vi "Create Groups.vi"(8 "error in (no error)":errorcluster, 10 "Framework Configuration":refnum<class "Framework Configuration.lvclass">, 11 "Framework in":refnum<class "Framework.lvclass">) -> (0 "error out":errorcluster, 2 "Transfer Groups":refnum<class "Transfer Group.lvclass">[](array[class]), 3 "Framework out":refnum<class "Framework.lvclass">)   [LabVIEW 2017, in "DSF Core.lvlib" / "Framework.lvclass"]
uses:
  Framework.lvclass
  Configuration/Core/Framework/Framework Configuration.lvclass
  Transfer Group/Transfer Group.lvclass
  Configuration/Core/Framework/Framework Configuration.lvclass/Framework Configuration.ctl
  Configuration/Core/Plugin/Plugin Configuration.lvclass/Plugin Configuration.ctl
  Configuration/Core/Thread/Thread Configuration.lvclass/Thread Configuration.ctl
  Buffer/Buffer.lvclass
  C:/Program Files (x86)/National Instruments/LabVIEW 2017/vi.lib/NI/Memory Manager/Classes/Pointer/Pointer.lvclass
  Configuration/Core/Group/Group Configuration.lvclass/Group Configuration.ctl
  <vilib>/NI/Memory Manager/Classes/Pointer/Pointer.lvclass/Pointer.ctl
  Transfer Group/Transfer Offsets.ctl
  <vilib>/NI/Memory Manager/Classes/Pointer/Set Size.vi
  <vilib>/NI/Memory Manager/Classes/Pointer/Set Address.vi
  <vilib>/NI/Memory Manager/Classes/Pointer/Check Null Pointer.vi
  <vilib>/NI/Memory Manager/Classes/Pointer/Set Internal.vi
  <vilib>/NI/Memory Manager/Classes/Pointer/Errors.vi
  <vilib>/NI/Memory Manager/Classes/Pointer/Null Pointer.vi
  <vilib>/NI/Memory Manager/Classes/Pointer/Is Null.vi
  <vilib>/NI/Memory Manager/Classes/Pointer/Create Error.vi
  <vilib>/NI/Memory Manager/Classes/Pointer/Get Address.vi
  <vilib>/NI/Memory Manager/Constants/Constants.vi
  <vilib>/NI/Memory Manager/Constants/Library Name.vi
  <vilib>/NI/Memory Manager/Classes/Pointer/Pointer Error Info.vi
  <vilib>/NI/Memory Manager/Constants/Pointer Class Name.vi
  <vilib>/NI/Memory Manager/VIs/New Error Cluster.vi
  <vilib>/NI/Memory Manager/VIs/New Error Cluster (512B).vi
  <vilib>/NI/Memory Manager/VIs/Set Error Status.vi
  <vilib>/NI/Memory Manager/VIs/Set Error Code.vi
  <vilib>/NI/Memory Manager/VIs/Set Error Source.vi
  <vilib>/NI/Memory Manager/VIs/Write String to Source.vi
  Configuration/Core/Group/Group Configuration.lvclass
  Configuration/Core/Transfer/Transfer Configuration.lvclass
  Configuration/Core/Plugin/Plugin Configuration.lvclass
  Configuration/Core/Thread/Thread Configuration.lvclass
  <vilib>/NI/Memory Manager/Classes/Pointer/Pointer.lvclass
  Buffers/Buffers.lvclass
  Transfer/Transfer.lvclass
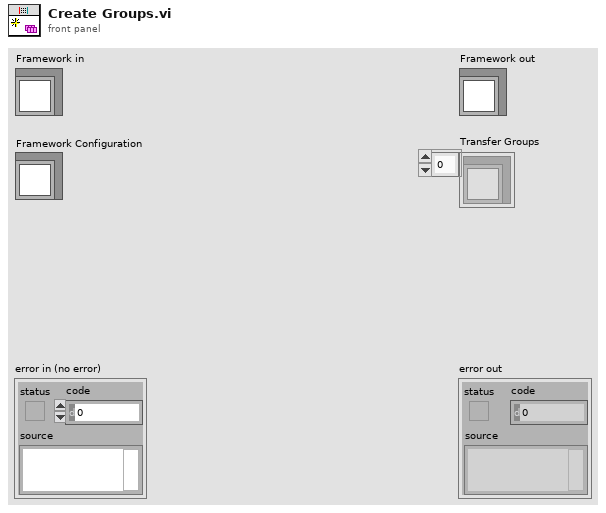
[diagram p1: front panel]
types:
  T1 = typedef "DSF Core.lvlib/Transfer Group.lvclass/Transfer Offsets.ctl" = cluster{"string offset":u64, "engine offset":u64}
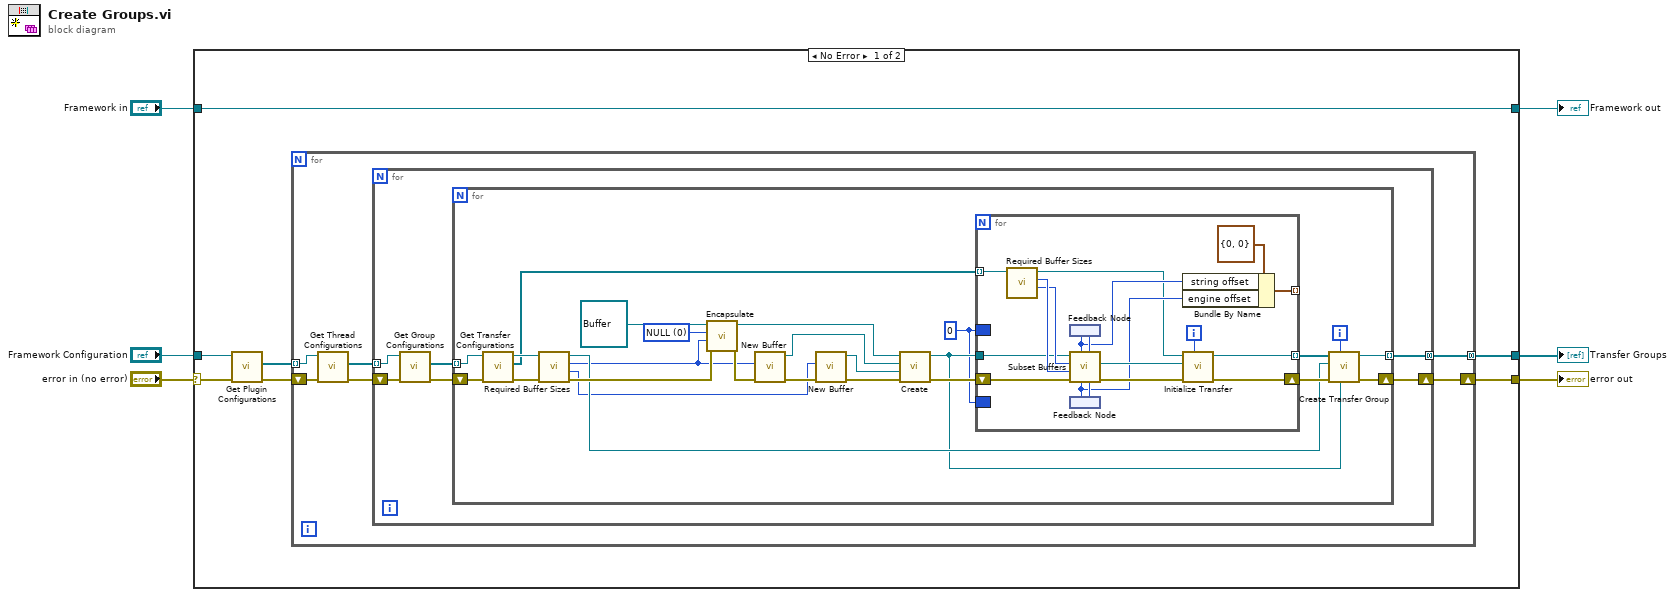
[diagram p0: block diagram]
diagram:
  n1 = case shown="No Error" "error in (no error)" {
    selector: "error in (no error)" -> [w9 w69]
    tunnel: [w8 w69] -> w5
    tunnel: [w7 w68] -> w3
    tunnel: "Framework in" -> [w7 w68]
    tunnel: "Framework Configuration" -> [w12 _]
    tunnel: [w10 _] -> w1
    frame No Error {
      n2 = call "Get Plugin Configurations.vi"("error in (no error)"=w9, "Framework Configuration in"=w12) -> ("error out"=w11:errorcluster, "Plugin Configurations"=w13:refnum<class "Plugin Configuration.lvclass">[])  [unwired: 7 in, 1 out]
      n3 = for {
        tunnel: w13 -> [w19] mode=indexing
        shift-right: [w14] -> w8
        shift-left: w11 -> [w17]
        tunnel: [w15] -> w10 mode=concatenating
        n4 = call "Get Thread Configurations.vi"("error in (no error)"=w17, "Plugin Configuration in"=w19) -> ("error out"=w16:errorcluster, "Thread Configurations"=w18:refnum<class "Thread Configuration.lvclass">[])  [unwired: 7 in, 1 out]
        n5 = for {
          tunnel: w18 -> [w25] mode=indexing
          shift-right: [w20] -> w14
          shift-left: w16 -> [w23]
          tunnel: [w21] -> w15 mode=concatenating
          n6 = call "Get Group Configurations.vi"("error in (no error)"=w23, "Thread Configuration in"=w25) -> ("error out"=w22:errorcluster, "Group Configurations"=w24:refnum<class "Group Configuration.lvclass">[])  [unwired: 7 in, 1 out]
          n7 = for {
            tunnel: w24 -> [w34] mode=indexing
            shift-right: [w47] -> w20
            shift-left: w22 -> [w35]
            tunnel: [w48] -> w21 mode=indexing
            i -> [w46]
            w43 = u64 0 items=["NULL"] ("Null")
            w26 = u64 0 ("inline buffer size")
            n8 = call "Get Transfer Configurations.vi"("error in (no error)"=w35, "Group Configuration in"=w34) -> ("error out"=w33:errorcluster, "Transfer Configurations"=w31:refnum<class "Transfer Configuration.lvclass">[], "Group Configuration out"=w32:refnum<class "Group Configuration.lvclass">)  [unwired: 7 in]
            n9 = call-dynamic "Required Buffer Sizes.vi"("error in (no error)"=w33, "Group Configuration in"=w32) -> ("error out"=w38:errorcluster, "string size"=w28:u64, "engine size"=w27:u64, "Group Configuration out"=w30:refnum<class "Group Configuration.lvclass">)  [unwired: 6 in]
            n10 = call <vilib>:"Encapsulate.vi"("error in (no error)"=w38, "size"=w27, "address"=w43, "Pointer type"=refnum<class "Buffer.lvclass"> refnum ("Inline Buffer (null)")) -> ("error out"=w37:errorcluster, "Pointer"=w39:refnum<class "Buffer.lvclass">)  [unwired: 6 in]
            n11 = call "New Buffer.vi"("error in (no error)"=w37, "buffer size"=w27) -> ("error out"=w45:errorcluster, "Buffer out"=w41:refnum<class "Buffer.lvclass">)  [unwired: 8 in]
            n12 = call "New Buffer.vi"("error in (no error)"=w45, "buffer size"=w28) -> ("error out"=w40:errorcluster, "Buffer out"=w44:refnum<class "Buffer.lvclass">)  [unwired: 8 in]
            n13 = call "Create.vi"("error in (no error)"=w40, "String Buffer (null)"=w44, "Async Buffer (null)"=w41, "Inline Buffer (null)"=w39) -> ("error out"=w36:errorcluster, "Buffers out"=w29:refnum<class "Buffers.lvclass">)  [unwired: 6 in]
            n14 = for {
              tunnel: [w67] -> w49 mode=indexing
              shift-right: [w66] -> w50
              shift-left: w36 -> [w64]
              border: w26 -> [_]
              border: w26 -> [_]
              tunnel: [w58] -> _ mode=indexing
              tunnel: w31 -> [w55] mode=indexing
              tunnel: w29 -> [w51]
              i -> [w65]
              n15 = call-dynamic "Required Buffer Sizes.vi"("Transfer Configuration in"=w55) -> ("string size"=w53:u64, "engine size"=w54:u64, "Transfer Configuration out"=w52:refnum<class "Transfer Configuration.lvclass">)  [unwired: 7 in, 1 out]
              n16 = feedback #1() -> (w57:u64)
              n17 = feedback #2() -> (w56:u64)
              n18 = call "Subset Buffers.vi"("engine buffer offset"=w56, "string buffer offset"=w57, "error in (no error)"=w64, "engine buffer size"=w54, "string buffer size"=w53, "Buffers in"=w51) -> ("error out"=w61:errorcluster, "subset Buffers"=w60:refnum<class "Buffers.lvclass">, "engine buffer offset +size"=w63:u64, "string buffer offset + size"=w62:u64)  [unwired: 1 in, 1 out]
              n19 = feedback-in #1(w62) -> ()
              n20 = feedback-in #2(w63) -> ()
              n21 = Bundle By Name(cluster=T1 {"string offset"=0, "engine offset"=0} ("offsets"), "string offset"=w57, "engine offset"=w56) -> (w58:T1)
              n22 = call "Initialize Transfer.vi"("id"=w65, "error in (no error)"=w61, "Buffers"=w60, "Transfer Configuration"=w52) -> ("error out"=w66:errorcluster, "Transfer out"=w67:refnum<class "Transfer.lvclass">)  [unwired: 6 in]
            }
            n23 = call "Create Transfer Group.vi"("Buffers"=w29, "id"=w46, "error in (no error)"=w50, "Group Configuration"=w30, "Transfers"=w49) -> ("error out"=w47:errorcluster, "Transfer Group out"=w48:refnum<class "Transfer Group.lvclass">)  [unwired: 5 in]
          }
        }
      }
    }
    frame Error {
    }
  }
  "error out" <- w5
  "Framework out" <- w3
  "Transfer Groups" <- w1
